vi "Test IV and Ic distribution V2.vi"() -> ()   [LabVIEW 2023]
uses:
  RT fast data.ctl
  <vilib>/LabVIEW Targets/FPGA/cRIO/shared/nicrio_ModuleControls/nicrio_cRIO-9775_RecordDataRates4ChansRing.ctl
  <vilib>/LabVIEW Targets/FPGA/cRIO/shared/nicrio_ModuleControls/nicrio_BasicConversionTime.ctl
  Ramps.ctl
  <resource>/objmgr/ni.dex.rc
  <vilib>/Analysis/NI_AALBase.lvlib
panel:
  out "Histogram Graph":T1(graph)={"X Values"=[0.276722412109375, 0.276944580078125, 0.277166748046875, 0.27738891601562504, 0.27761108398437506, 0.2778332519531251, 0.2780554199218751, 0.2782775878906251, 0.27849975585937514, 0.27872192382812516, 0.2789440917968752, 0.2791662597656252, 0.2793884277343752, 0.27961059570312524, 0.27983276367187526, 0.2800549316406253, 0.2802770996093753, 0.2804992675781253, 0.28072143554687534, 0.28094360351562536, 0.2811657714843754, 0.2813879394531254, 0.2816101074218754, 0.28183227539062544, 0.28205444335937546, 0.2822766113281255, 0.2824987792968755, 0.2827209472656255, 0.28294311523437554, 0.28316528320312556, 0.2833874511718756, 0.2836096191406256, 0.2838317871093756, 0.28405395507812564, 0.28427612304687566, 0.2844982910156257, 0.2847204589843757, 0.2849426269531257, 0.28516479492187574, 0.28538696289062576, 0.2856091308593758, 0.2858312988281258, 0.2860534667968758, 0.28627563476562584, 0.28649780273437586, 0.2867199707031259, 0.2869421386718759, 0.2871643066406259, 0.28738647460937594, 0.28760864257812596, 0.287830810546876, 0.288052978515626, 0.288275146484376, 0.28849731445312604, 0.28871948242187606, 0.2889416503906261, 0.2891638183593761, 0.2893859863281261, 0.28960815429687614, 0.28983032226562616, 0.2900524902343762, 0.2902746582031262, 0.2904968261718762, 0.29071899414062624, 0.29094116210937626, 0.2911633300781263, 0.2913854980468763, 0.2916076660156263, 0.29182983398437634, 0.29205200195312636, 0.2922741699218764, 0.2924963378906264, 0.2927185058593764, 0.29294067382812644, 0.29316284179687646, 0.2933850097656265, 0.2936071777343765, 0.2938293457031265, 0.29405151367187654, 0.29427368164062656, 0.2944958496093766, 0.2947180175781266, 0.2949401855468766, 0.29516235351562664, 0.29538452148437666, 0.2956066894531267, 0.2958288574218767, 0.2960510253906267, 0.29627319335937674, 0.29649536132812676, 0.2967175292968768, 0.2969396972656268, 0.2971618652343768, 0.29738403320312684, 0.29760620117187686, 0.2978283691406269, 0.2980505371093769, 0.2982727050781269, 0.29849487304687694, 0.29871704101562696], "Histogram: h(x)"=[1, 0, 0, 0, 0, 0, 0, 0, 0, 0, 0, 0, 3, 0, 0, 0, 0, 0, 0, 0, 0, 0, 0, 0, 0, 8, 0, 0, 0, 0, 7, 0, 0, 0, 0, 0, 0, 16, 0, 0, 0, 0, 0, 8, 0, 0, 0, 0, 0, 20, 0, 0, 0, 0, 0, 0, 10, 0, 0, 0, 0, 0, 14, 0, 0, 0, 0, 0, 3, 0, 0, 0, 0, 0, 5, 0, 0, 0, 0, 0, 0, 4, 0, 0, 0, 0, 0, 0, 0, 0, 0, 0, 0, 0, 0, 0, 0, 0, 0, 1]}
  out "PCreaderV":refnum<k21>="PCreaderV"
  out "PC para writer":refnum<k21>="PCwriter"
  out "PCreaderI":refnum<k21>="PCreaderI"
  out "DAQ_AI_Reader endpoint":refnum<k21>="DAQ_AI_Reader"
  out "DAQ_CMD_Writer endpoint":refnum<k21>="DAQ_CMD_Writer"
  out "vi reference":refnum<vi>
  out "application reference":refnum<vi>
  in  "Tab Control":enum32{"IV", "Ic"}(tab)=enum."Ic"
  in  "IV parameters":T2={"Records Num"=1, "AI Trigger Configuration"={"Trigger Slope"=enum."Positive", "Trigger Level"=0.89990234375, "Hystesis Value"=0.0, "AI Channel"=0}, "Record PreTrigger Samples"=1, "Record Samples"=5000, "Ic Cut off or curve"=FALSE, "Record Data Rate"=200, "Wait before trigger us"=1, "Cutoff delay usec"=1, "Timing Mode"=enum."High Resolution", "Trigger length ticks"=1, "Timeout"=-1, "Ramps"={"Amp"=1.0, "Delay time 10us"=1, "Ramp1 time 10us"=1000, "Ramp2 time 10us"=2000, "Ramp3 time 10us"=1000, "End time 10us"=1}} {"Record Data Rate" items=["20.000 MS/s (NI 9775)"=1, "10.00 MS/s (NI 9775)"=2, "6.667 MS/s (NI 9775)"=3, "5.000 MS/s (NI 9775)"=4, "2.500 MS/s (NI 9775)"=8, "1.667 MS/s (NI 9775)"=12, "1.250 MS/s (NI 9775)"=16, "1.000 MS/s (NI 9775)"=20, "833.333 KS/s (NI 9775)"=24, "714.286 KS/s (NI 9775)"=28, "625.000 KS/s (NI 9775)"=32, "555.556 KS/s (NI 9775)"=36, "500.000 KS/s (NI 9775)"=40, "454.545 KS/s (NI 9775)"=44, "416.667 KS/s (NI 9775)"=48, "384.615 KS/s (NI 9775)"=52, "357.143 KS/s (NI 9775)"=56, "333.333 KS/s (NI 9775)"=60, "312.500 KS/s (NI 9775)"=64, "294.118 KS/s (NI 9775)"=68, "277.778 KS/s (NI 9775)"=72, "263.158 KS/s (NI 9775)"=76, "250.000 KS/s (NI 9775)"=80, "238.095 KS/s (NI 9775)"=84, "227.273 KS/s (NI 9775)"=88, "217.391 KS/s (NI 9775)"=92, "208.333 KS/s (NI 9775)"=96, "200.000 KS/s (NI 9775)"=100, "192.308 KS/s (NI 9775)"=104, "185.185 KS/s (NI 9775)"=108, "178.571 KS/s (NI 9775)"=112, "172.414 KS/s (NI 9775)"=116, "166.667 KS/s (NI 9775)"=120, "161.290 KS/s (NI 9775)"=124, "156.250 KS/s (NI 9775)"=128, "151.515 KS/s (NI 9775)"=132, "147.059 KS/s (NI 9775)"=136, "142.857 KS/s (NI 9775)"=140, "138.889 KS/s (NI 9775)"=144, "135.135 KS/s (NI 9775)"=148, "131.579 KS/s (NI 9775)"=152, "128.205 KS/s (NI 9775)"=156, "125.000 KS/s (NI 9775)"=160, "121.951 KS/s (NI 9775)"=164, "119.048 KS/s (NI 9775)"=168, "116.279 KS/s (NI 9775)"=172, "113.636 KS/s (NI 9775)"=176, "111.111 KS/s (NI 9775)"=180, "108.696 KS/s (NI 9775)"=184, "106.383 KS/s (NI 9775)"=188, "104.167 KS/s (NI 9775)"=192, "102.041 KS/s (NI 9775)"=196, "100.000 KS/s (NI 9775)"=200, "50.000 KS/s (NI 9775)"=400, "33.333 KS/s (NI 9775)"=600, "25.000 KS/s (NI 9775)"=800, "20.000 KS/s (NI 9775)"=1000, "16.667 KS/s (NI 9775)"=1200, "14.286 KS/s (NI 9775)"=1400, "12.500 KS/s (NI 9775)"=1600, "11.111 KS/s (NI 9775)"=1800, "10.000 KS/s (NI 9775)"=2000, "9.091 KS/s (NI 9775)"=2200, "8.333 KS/s (NI 9775)"=2400, "7.692 KS/s (NI 9775)"=2600, "7.143 KS/s (NI 9775)"=2800, "6.667 KS/s (NI 9775)"=3000, "6.250 KS/s (NI 9775)"=3200, "5.882 KS/s (NI 9775)"=3400, "5.556 KS/s (NI 9775)"=3600, "5.000 KS/s (NI 9775)"=4000, "4.762 KS/s (NI 9775)"=4200, "4.545 KS/s (NI 9775)"=4400, "4.348 KS/s (NI 9775)"=4600, "4.167 KS/s (NI 9775)"=4800, "4.000 KS/s (NI 9775)"=5000, "3.846 KS/s (NI 9775)"=5200, "3.571 KS/s (NI 9775)"=5600, "3.333 KS/s (NI 9775)"=6000, "3.125 KS/s (NI 9775)"=6400, "2.941 KS/s (NI 9775)"=6800, "2.778 KS/s (NI 9775)"=7200, "2.632 KS/s (NI 9775)"=7600, "2.500 KS/s (NI 9775)"=8000, "2.381 KS/s (NI 9775)"=8400, "2.273 KS/s (NI 9775)"=8800, "2.174 KS/s (NI 9775)"=9200, "2.083 KS/s (NI 9775)"=9600, "2.000 KS/s (NI 9775)"=10000, "1.923 KS/s (NI 9775)"=10400, "1.852 KS/s (NI 9775)"=10800, "1.786 KS/s (NI 9775)"=11200, "1.724 KS/s (NI 9775)"=11600, "1.667 KS/s (NI 9775)"=12000, "1.613 KS/s (NI 9775)"=12400, "1.563 KS/s (NI 9775)"=12800, "1.515 KS/s (NI 9775)"=13200, "1.471 KS/s (NI 9775)"=13600, "1.429 KS/s (NI 9775)"=14000, "1.389 KS/s (NI 9775)"=14400, "1.351 KS/s (NI 9775)"=14800, "1.316 KS/s (NI 9775)"=15200, "1.282 KS/s (NI 9775)"=15600, "1.250 KS/s (NI 9775)"=16000, "1.220 KS/s (NI 9775)"=16400, "1.190 KS/s (NI 9775)"=16800, "1.163 KS/s (NI 9775)"=17200, "1.136 KS/s (NI 9775)"=17600, "1.111 KS/s (NI 9775)"=18000, "1.087 KS/s (NI 9775)"=18400, "1.064 KS/s (NI 9775)"=18800, "1.042 KS/s (NI 9775)"=19200, "1.020 KS/s (NI 9775)"=19600, "1.000 KS/s (NI 9775)"=20000, "0.980 KS/s (NI 9775)"=20400, "0.962 KS/s (NI 9775)"=20800, "0.943 KS/s (NI 9775)"=21200, "0.926 KS/s (NI 9775)"=21600, "0.909 KS/s (NI 9775)"=22000, "0.893 KS/s (NI 9775)"=22400, "0.877 KS/s (NI 9775)"=22800, "0.862 KS/s (NI 9775)"=23200, "0.847 KS/s (NI 9775)"=23600, "0.833 KS/s (NI 9775)"=24000, "0.820 KS/s (NI 9775)"=24400, "0.806 KS/s (NI 9775)"=24800, "0.794 KS/s (NI 9775)"=25200, "0.781 KS/s (NI 9775)"=25600, "0.694 KS/s (NI 9775)"=28800, "0.625 KS/s (NI 9775)"=32000, "0.568 KS/s (NI 9775)"=35200, "0.521 KS/s (NI 9775)"=38400, "0.446 KS/s (NI 9775)"=44800, "0.391 KS/s (NI 9775)"=51200, "0.347 KS/s (NI 9775)"=57600, "0.313 KS/s (NI 9775)"=64000]}
  in  "Ic parameters":T2={"Records Num"=100, "AI Trigger Configuration"={"Trigger Slope"=enum."Positive", "Trigger Level"=1.0, "Hystesis Value"=0.0, "AI Channel"=0}, "Record PreTrigger Samples"=1, "Record Samples"=16, "Ic Cut off or curve"=TRUE, "Record Data Rate"=1, "Wait before trigger us"=1, "Cutoff delay usec"=1, "Timing Mode"=enum."High Resolution", "Trigger length ticks"=1, "Timeout"=-1, "Ramps"={"Amp"=1.0, "Delay time 10us"=1, "Ramp1 time 10us"=1000, "Ramp2 time 10us"=2000, "Ramp3 time 10us"=1000, "End time 10us"=1}} {"Record Data Rate" items=["20.000 MS/s (NI 9775)"=1, "10.00 MS/s (NI 9775)"=2, "6.667 MS/s (NI 9775)"=3, "5.000 MS/s (NI 9775)"=4, "2.500 MS/s (NI 9775)"=8, "1.667 MS/s (NI 9775)"=12, "1.250 MS/s (NI 9775)"=16, "1.000 MS/s (NI 9775)"=20, "833.333 KS/s (NI 9775)"=24, "714.286 KS/s (NI 9775)"=28, "625.000 KS/s (NI 9775)"=32, "555.556 KS/s (NI 9775)"=36, "500.000 KS/s (NI 9775)"=40, "454.545 KS/s (NI 9775)"=44, "416.667 KS/s (NI 9775)"=48, "384.615 KS/s (NI 9775)"=52, "357.143 KS/s (NI 9775)"=56, "333.333 KS/s (NI 9775)"=60, "312.500 KS/s (NI 9775)"=64, "294.118 KS/s (NI 9775)"=68, "277.778 KS/s (NI 9775)"=72, "263.158 KS/s (NI 9775)"=76, "250.000 KS/s (NI 9775)"=80, "238.095 KS/s (NI 9775)"=84, "227.273 KS/s (NI 9775)"=88, "217.391 KS/s (NI 9775)"=92, "208.333 KS/s (NI 9775)"=96, "200.000 KS/s (NI 9775)"=100, "192.308 KS/s (NI 9775)"=104, "185.185 KS/s (NI 9775)"=108, "178.571 KS/s (NI 9775)"=112, "172.414 KS/s (NI 9775)"=116, "166.667 KS/s (NI 9775)"=120, "161.290 KS/s (NI 9775)"=124, "156.250 KS/s (NI 9775)"=128, "151.515 KS/s (NI 9775)"=132, "147.059 KS/s (NI 9775)"=136, "142.857 KS/s (NI 9775)"=140, "138.889 KS/s (NI 9775)"=144, "135.135 KS/s (NI 9775)"=148, "131.579 KS/s (NI 9775)"=152, "128.205 KS/s (NI 9775)"=156, "125.000 KS/s (NI 9775)"=160, "121.951 KS/s (NI 9775)"=164, "119.048 KS/s (NI 9775)"=168, "116.279 KS/s (NI 9775)"=172, "113.636 KS/s (NI 9775)"=176, "111.111 KS/s (NI 9775)"=180, "108.696 KS/s (NI 9775)"=184, "106.383 KS/s (NI 9775)"=188, "104.167 KS/s (NI 9775)"=192, "102.041 KS/s (NI 9775)"=196, "100.000 KS/s (NI 9775)"=200, "50.000 KS/s (NI 9775)"=400, "33.333 KS/s (NI 9775)"=600, "25.000 KS/s (NI 9775)"=800, "20.000 KS/s (NI 9775)"=1000, "16.667 KS/s (NI 9775)"=1200, "14.286 KS/s (NI 9775)"=1400, "12.500 KS/s (NI 9775)"=1600, "11.111 KS/s (NI 9775)"=1800, "10.000 KS/s (NI 9775)"=2000, "9.091 KS/s (NI 9775)"=2200, "8.333 KS/s (NI 9775)"=2400, "7.692 KS/s (NI 9775)"=2600, "7.143 KS/s (NI 9775)"=2800, "6.667 KS/s (NI 9775)"=3000, "6.250 KS/s (NI 9775)"=3200, "5.882 KS/s (NI 9775)"=3400, "5.556 KS/s (NI 9775)"=3600, "5.000 KS/s (NI 9775)"=4000, "4.762 KS/s (NI 9775)"=4200, "4.545 KS/s (NI 9775)"=4400, "4.348 KS/s (NI 9775)"=4600, "4.167 KS/s (NI 9775)"=4800, "4.000 KS/s (NI 9775)"=5000, "3.846 KS/s (NI 9775)"=5200, "3.571 KS/s (NI 9775)"=5600, "3.333 KS/s (NI 9775)"=6000, "3.125 KS/s (NI 9775)"=6400, "2.941 KS/s (NI 9775)"=6800, "2.778 KS/s (NI 9775)"=7200, "2.632 KS/s (NI 9775)"=7600, "2.500 KS/s (NI 9775)"=8000, "2.381 KS/s (NI 9775)"=8400, "2.273 KS/s (NI 9775)"=8800, "2.174 KS/s (NI 9775)"=9200, "2.083 KS/s (NI 9775)"=9600, "2.000 KS/s (NI 9775)"=10000, "1.923 KS/s (NI 9775)"=10400, "1.852 KS/s (NI 9775)"=10800, "1.786 KS/s (NI 9775)"=11200, "1.724 KS/s (NI 9775)"=11600, "1.667 KS/s (NI 9775)"=12000, "1.613 KS/s (NI 9775)"=12400, "1.563 KS/s (NI 9775)"=12800, "1.515 KS/s (NI 9775)"=13200, "1.471 KS/s (NI 9775)"=13600, "1.429 KS/s (NI 9775)"=14000, "1.389 KS/s (NI 9775)"=14400, "1.351 KS/s (NI 9775)"=14800, "1.316 KS/s (NI 9775)"=15200, "1.282 KS/s (NI 9775)"=15600, "1.250 KS/s (NI 9775)"=16000, "1.220 KS/s (NI 9775)"=16400, "1.190 KS/s (NI 9775)"=16800, "1.163 KS/s (NI 9775)"=17200, "1.136 KS/s (NI 9775)"=17600, "1.111 KS/s (NI 9775)"=18000, "1.087 KS/s (NI 9775)"=18400, "1.064 KS/s (NI 9775)"=18800, "1.042 KS/s (NI 9775)"=19200, "1.020 KS/s (NI 9775)"=19600, "1.000 KS/s (NI 9775)"=20000, "0.980 KS/s (NI 9775)"=20400, "0.962 KS/s (NI 9775)"=20800, "0.943 KS/s (NI 9775)"=21200, "0.926 KS/s (NI 9775)"=21600, "0.909 KS/s (NI 9775)"=22000, "0.893 KS/s (NI 9775)"=22400, "0.877 KS/s (NI 9775)"=22800, "0.862 KS/s (NI 9775)"=23200, "0.847 KS/s (NI 9775)"=23600, "0.833 KS/s (NI 9775)"=24000, "0.820 KS/s (NI 9775)"=24400, "0.806 KS/s (NI 9775)"=24800, "0.794 KS/s (NI 9775)"=25200, "0.781 KS/s (NI 9775)"=25600, "0.694 KS/s (NI 9775)"=28800, "0.625 KS/s (NI 9775)"=32000, "0.568 KS/s (NI 9775)"=35200, "0.521 KS/s (NI 9775)"=38400, "0.446 KS/s (NI 9775)"=44800, "0.391 KS/s (NI 9775)"=51200, "0.347 KS/s (NI 9775)"=57600, "0.313 KS/s (NI 9775)"=64000]}
  in  "IV length":i32=2000
  in  "IV points start":i32=1000
  out "Time to Init ms":u32=879
  out "Start time ms":u32=1037372149
  in  "Wire resistance":dbl
  in  "Read point":i32=1
  out "Done":bool
  out "Array":dbl[](array[numeric])=[0.286376953125, 0.29052734375, 0.293212890625, 0.283447265625, 0.2890625, 0.28759765625, 0.28759765625, 0.294677734375, 0.28759765625, 0.29052734375, 0.276611328125, 0.284912109375, 0.286376953125, 0.28759765625, 0.28759765625, 0.283447265625, 0.286376953125, 0.279296875, 0.29052734375, 0.294677734375, 0.2890625, 0.284912109375, 0.2822265625, 0.2890625, 0.2890625, 0.2890625, 0.284912109375, 0.2822265625, 0.284912109375, 0.29052734375, 0.29052734375, 0.284912109375, 0.284912109375, 0.284912109375, 0.283447265625, 0.284912109375, 0.28759765625, 0.284912109375, 0.28759765625, 0.293212890625, 0.28759765625, 0.29052734375, 0.29052734375, 0.286376953125, 0.286376953125, 0.29052734375, 0.29052734375, 0.283447265625, 0.28759765625, 0.2822265625, 0.2890625, 0.291748046875, 0.279296875, 0.284912109375, 0.2822265625, 0.286376953125, 0.2822265625, 0.28759765625, 0.2890625, 0.284912109375, 0.2890625, 0.283447265625, 0.293212890625, 0.291748046875, 0.28759765625, 0.28759765625, 0.28759765625, 0.293212890625, 0.284912109375, 0.279296875, 0.28759765625, 0.294677734375, 0.28759765625, 0.28759765625, 0.29052734375, 0.284912109375, 0.298828125, 0.28759765625, 0.29052734375, 0.29052734375, 0.283447265625, 0.284912109375, 0.286376953125, 0.294677734375, 0.2822265625, 0.286376953125, 0.2822265625, 0.284912109375, 0.2890625, 0.2822265625, 0.28759765625, 0.283447265625, 0.29052734375, 0.29052734375, 0.291748046875, 0.284912109375, 0.2890625, 0.293212890625, 0.28759765625, 0.28759765625]
  out "XY Graph":cluster{"Y":dbl[], "Y":dbl[]}[](graph)
  in  "Data buffer size":i32=1000
  out "error out":errorcluster
  in  "cRIO IP":string="//172.22.11.2"
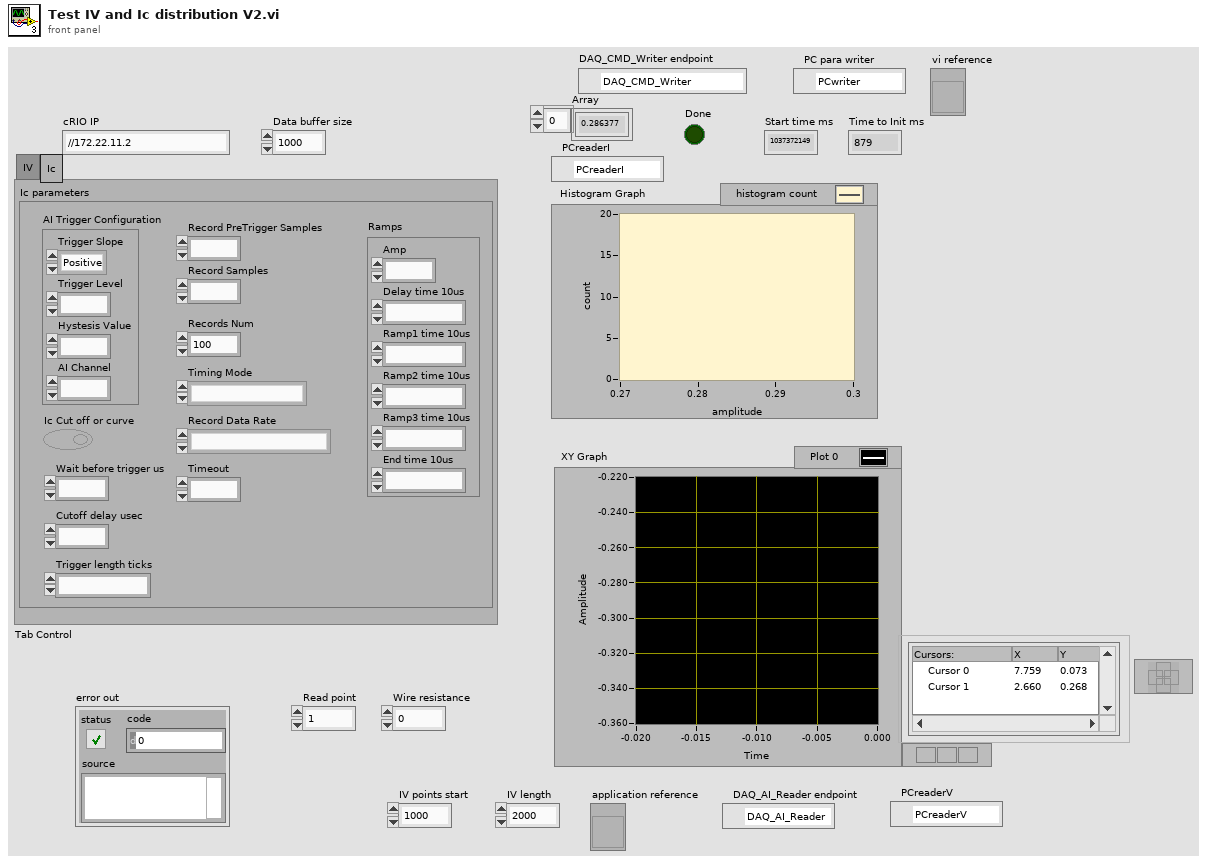
[diagram p1: front panel]
types:
  T1 = cluster{"X Values":dbl[], "Histogram: h(x)":i32[]}
  T2 = typedef "RT fast data.ctl" = cluster{"Records Num":i32, "AI Trigger Configuration":cluster{"Trigger Slope":enum8{"Positive", "Negative"}, "Trigger Level":fxp<+/-,17,5>, "Hystesis Value":fxp<+,16,4>, "AI Channel":u8}, "Record PreTrigger Samples":u32, "Record Samples":u32, "Ic Cut off or curve":bool, "Record Data Rate":T3, "Wait before trigger us":u32, "Cutoff delay usec":u32, "Timing Mode":T4, "Trigger length ticks":u32, "Timeout":i32, "Ramps":T5}
  T3 = typedef "nicrio_cRIO-9775_RecordDataRates4ChansRing.ctl" = u16
  T4 = typedef "nicrio_BasicConversionTime.ctl" = enum8{"High Speed", "High Resolution"}
  T5 = typedef "Ramps.ctl" = cluster{"Amp":fxp<+/-,20,5>, "Delay time 10us":i32, "Ramp1 time 10us":i32, "Ramp2 time 10us":i32, "Ramp3 time 10us":i32, "End time 10us":i32}
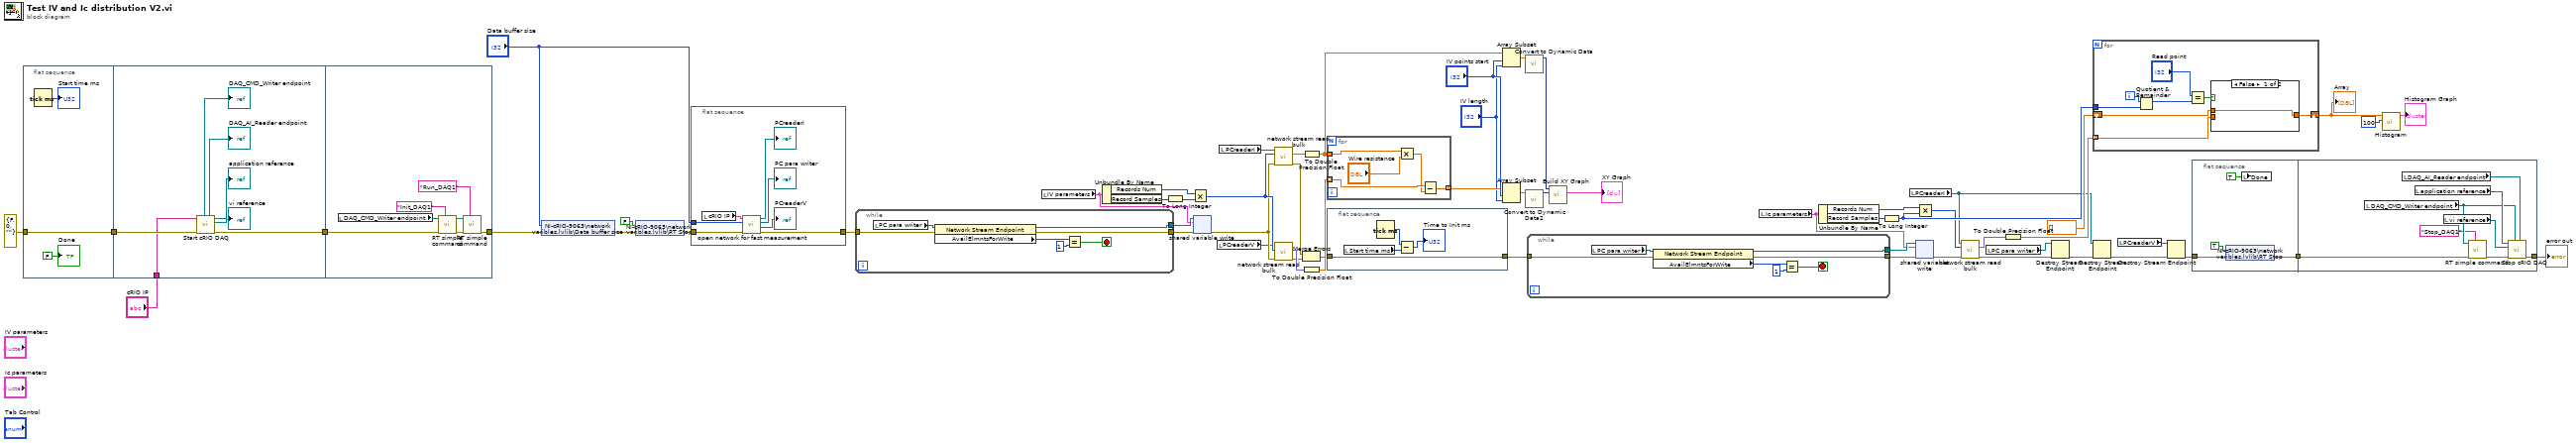
[diagram p0: block diagram]
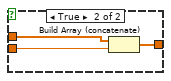
[diagram p2: hidden frame]
diagram:
  n1 = flat-sequence {
    tunnel: errorcluster {"status"=FALSE, "code"=0, "source"=""} ("error in (no error)") -> [w61]
    tunnel: [w61] -> w13
    tunnel: w13 -> [w65]
    tunnel: "cRIO IP" -> [w63]
    tunnel: [w64] -> w2
    tunnel: [w71] -> w12
    tunnel: w2 -> [w76]
    frame #0 {
      n2 = Tick Count (ms)() -> (millisecond timer value=→"Start time ms":u32)
      "Done" <- FALSE ("Done")
    }
    frame #1 {
      n3 = call "Start cRIO DAQ.vi"("error in (no error)"=w65, "cRIO IP"=w63) -> ("error out"=w64:errorcluster, "vi reference"=→"vi reference":refnum<vi>, "application reference"=→"application reference":refnum<vi>, "DAQ_AI_Reader endpoint"=→"DAQ_AI_Reader endpoint":refnum<k21>, "DAQ_CMD_Writer endpoint"=→"DAQ_CMD_Writer endpoint":refnum<k21>)  [unwired: 5 in]
    }
    frame #2 {
      n4 = local read "DAQ_CMD_Writer endpoint"() -> (w75:refnum<k21>)
      n5 = call "RT simple command.vi"("Command"="Init_DAQ1", "error in (no error)"=w76, "DAQ_CMD_Writer endpoint"=w75) -> ("error out"=w73:errorcluster, "DAQ_CMD_Writer endpoint out"=w72:refnum<k21>)  [unwired: 7 in]
      n6 = call "RT simple command.vi"("Command"="Run_DAQ1", "error in (no error)"=w73, "DAQ_CMD_Writer endpoint"=w72) -> ("error out"=w71:errorcluster)  [unwired: 7 in, 1 out]
    }
  }
  n7 = shared-variable "NI-cRIO-9063\\network varibles.lvlib\\Data buffer size"("Data buffer size", error in=w12) -> (error out=w56:errorcluster)
  n8 = shared-variable "NI-cRIO-9063\\network varibles.lvlib\\RT Stop"(FALSE ("RT Stop"), error in=w56) -> (error out=w11:errorcluster)
  n9 = flat-sequence {
    tunnel: w11 -> [w83]
    tunnel: "Data buffer size" -> [w82]
    tunnel: [w81] -> w8
    frame #0 {
      n10 = local read "cRIO IP"() -> (w77:string)
      n11 = call "open network for fast measurement.vi"("error in (no error)"=w83, "Data buffer size"=w82, "cRIO IP"=w77) -> ("error out"=w81:errorcluster, "PCreaderV"=→"PCreaderV":refnum<k21>, "PC para writer"=→"PC para writer":refnum<k21>, "PCreaderI"=→"PCreaderI":refnum<k21>)  [unwired: 5 in]
    }
  }
  n12 = while {
    tunnel: w8 -> [w90]
    tunnel: [w86] -> w58
    tunnel: [w85] -> w34
    stop <- w87 stop-if-true
    n13 = local read "PC para writer"() -> (w84:refnum<k21>)
    n14 = property class="Network Stream Endpoint"(reference=w84, error in=w90) -> (reference out=w86:refnum<k21>, error out=w85:errorcluster, "AvailElmntsForWrite"=w89:i32)
    n15 = Equal?(x=w89, y=1) -> (x = y?=w87:bool)
  }
  n16 = local read "IV parameters"() -> (w45:T2)
  n17 = Unbundle By Name(w45) -> ("Records Num"=w44:i32, "Record Samples"=w43:u32)
  n18 = To Long Integer(number=w43) -> (32bit integer=w42:i32)
  n19 = Multiply(x=w44, y=w42) -> (x*y=w29:i32)
  n20 = shared-variable-write(w58, w34, w45) -> (w22:errorcluster)  [unwired: 1 in, 2 out]
  n21 = local read "PCreaderV"() -> (w5:refnum<k21>)
  n22 = local read "PCreaderI"() -> (w6:refnum<k21>)
  n23 = call "network stream read bulk.vi"("endpoint in"=w6, "Data num"=w29, "error in (no error)"=w22) -> ("Data"=w31:fxp<+/-,17,5>[], "error out"=w28:errorcluster)  [unwired: 5 in, 1 out]
  n24 = call "network stream read bulk.vi"("endpoint in"=w5, "Data num"=w29, "error in (no error)"=w22) -> ("Data"=w30:fxp<+/-,17,5>[], "error out"=w27:errorcluster)  [unwired: 5 in, 1 out]
  n25 = Merge Errors(w28, w27) -> (w33:errorcluster)
  n26 = To Double Precision Float(number=w30) -> (double precision float=w35:dbl[])
  n27 = To Double Precision Float(number=w31) -> (double precision float=w20:dbl[])
  n28 = for {
    tunnel: w35 -> [w95] mode=indexing
    tunnel: w20 -> [w93] mode=indexing
    tunnel: [w91] -> w18 mode=indexing
    n29 = Multiply(x=w93, y="Wire resistance") -> (x*y=w92:dbl)
    n30 = Subtract(x=w95, y=w92) -> (x-y=w91:dbl)
  }
  n31 = flat-sequence {
    tunnel: w33 -> [w96]
    tunnel: [w96] -> w32
    frame #0 {
      n32 = local read "Start time ms"() -> (w98:u32)
      n33 = Tick Count (ms)() -> (millisecond timer value=w99:u32)
      n34 = Subtract(x=w99, y=w98) -> (x-y=→"Time to Init ms":u32)
    }
  }
  n35 = Array Subset(array=w20, index="IV points start", length="IV length") -> (w19:dbl[])
  n36 = Array Subset(array=w18, index="IV points start", length="IV length") -> (w17:dbl[])
  n37 = call "Convert to Dynamic Data"("Array"=w19) -> ("Dynamic Data Type"=w50:dynamicdata)  [unwired: 3 in]
  n38 = call "Convert to Dynamic Data2"("Array"=w17) -> ("Dynamic Data Type"=w49:dynamicdata)  [unwired: 3 in]
  n39 = while {
    tunnel: w32 -> [w104]
    tunnel: [w102] -> w53
    tunnel: [w101] -> w52
    stop <- w103 stop-if-true
    n40 = local read "PC para writer"() -> (w100:refnum<k21>)
    n41 = property class="Network Stream Endpoint"(reference=w100, error in=w104) -> (reference out=w102:refnum<k21>, error out=w101:errorcluster, "AvailElmntsForWrite"=w106:i32)
    n42 = Equal?(x=w106, y=1) -> (x = y?=w103:bool)
  }
  n43 = call "Build XY Graph"("Y Input"=w49, "X Input"=w50) -> ("XY Graph"=→"XY Graph":cluster{"X":dbl[], "Y":dbl[]}[])  [unwired: 8 in, 1 out]
  n44 = local read "Ic parameters"() -> (w48:T2)
  n45 = Unbundle By Name(w48) -> ("Records Num"=w47:i32, "Record Samples"=w46:u32)
  n46 = To Long Integer(number=w46) -> (32bit integer=w39:i32)
  n47 = local read "PCreaderI"() -> (w4:refnum<k21>)
  n48 = shared-variable-write(w53, w52, w48) -> (w25:errorcluster)  [unwired: 1 in, 2 out]
  n49 = Multiply(x=w47, y=w39) -> (x*y=w23:i32)
  n50 = call "network stream read bulk.vi"("endpoint in"=w4, "Data num"=w23, "error in (no error)"=w25) -> ("Data"=w26:fxp<+/-,17,5>[], "error out"=w24:errorcluster)  [unwired: 5 in, 1 out]
  n51 = local read "PC para writer"() -> (w7:refnum<k21>)
  n52 = To Double Precision Float(number=w26) -> (double precision float=w40:dbl[])
  n53 = Destroy Stream Endpoint(8:w24, 11:w7) -> (0:w57:errorcluster)
  n54 = for {
    tunnel: w40 -> [w108] mode=indexing
    tunnel: w39 -> [w114]
    shift-right: [w110] -> w37
    shift-left: dbl[] [] -> [w109]
    i -> [w113]
    n55 = Quotient & Remainder(x=w113, y=w114) -> (x-y*floor(x/y)=w112:i32)  [unwired: 1 out]
    n56 = Equal?(x="Read point", y=w112) -> (x = y?=w107:bool)
    n57 = case shown="False" w107 {
      tunnel: [w115 w118] -> w110
      tunnel: w109 -> [w115 w117]
      tunnel: w108 -> [_ w116]
      frame False {
      }
      frame True {
        n58 = Build Array (concatenate)(w117, w116) -> (w118:dbl[])
      }
    }
  }
  "Array" <- w37
  n59 = Destroy Stream Endpoint(8:w57, 11:w4) -> (0:w55:errorcluster)
  n60 = local read "PCreaderV"() -> (w3:refnum<k21>)
  n61 = Destroy Stream Endpoint(8:w55, 11:w3) -> (0:w54:errorcluster)
  n62 = flat-sequence {
    tunnel: w54 -> [w121]
    tunnel: [w122] -> w15
    tunnel: w15 -> [w126]
    tunnel: [w127] -> w14
    frame #0 {
      n63 = shared-variable "NI-cRIO-9063\\network varibles.lvlib\\RT Stop"(TRUE ("RT Stop"), error in=w121) -> (error out=w122:errorcluster)
      n64 = local write "Done"(TRUE ("Done")) -> ()
    }
    frame #1 {
      n65 = local read "DAQ_CMD_Writer endpoint"() -> (w124:refnum<k21>)
      n66 = local read "DAQ_AI_Reader endpoint"() -> (w130:refnum<k21>)
      n67 = local read "application reference"() -> (w128:refnum<vi>)
      n68 = local read "vi reference"() -> (w129:refnum<vi>)
      n69 = call "RT simple command.vi"("Command"="Stop_DAQ1", "error in (no error)"=w126, "DAQ_CMD_Writer endpoint"=w124) -> ("error out"=w125:errorcluster)  [unwired: 7 in, 1 out]
      n70 = call "Stop cRIO DAQ.vi"("DAQ_AI_Reader endpoint"=w130, "DAQ_CMD_Writer endpoint"=w124, "error in (no error)"=w125, "VI reference"=w129, "application reference"=w128) -> ("error out"=w127:errorcluster)  [unwired: 6 in]
    }
  }
  n71 = call <vilib>:"Histogram.vi"("intervals"=100, "X"=w37) -> ("Histogram Graph"=→"Histogram Graph":T1)  [unwired: 6 in, 3 out]
  "error out" <- w14
